vi "CLC_GEN3_L2_InPhaseCal.vi"() -> ()   [LabVIEW 2023, in "Clover_Cell.lvlib"]
uses:
  Clover_Cell.lvlib
  lib/Anritsu Signal Analyzer Series/Anritsu Signal Analyzer Series.lvlib
  lib/ELTA/ELTA.lvlib
  <vilib>/Utility/file.llb/Write Delimited Spreadsheet (DBL).vi
  <vilib>/Utility/file.llb/Write Delimited Spreadsheet (string).vi
panel:
  out "Check Ref. Ch.":i32[][](array[numeric])
  in  "Dual_Ch.???":bool=TRUE
  in  "Single_Channel_Phase_Sweep":bool
  in  "Polarity":u16(ring) items=["H", "V"]
  in  "AvgTimes":i32=3
  in  "TRXmode":u16(ring)=1 items=["Rx"=2, "Tx"=1]
  in  "CenterFreq(GHz)":dbl=27.0
  in  "VISA resource name":refnum<visa-resource-name>="TCPIP0::192.168.100.202::hislip0::INSTR"
  out "Channel":i32=63
  out "Operating \nChannel(s)":bool[][](array[boolean])
  out "FileNAME_Dual":string
  out "FileNAME_Single":string
  out "PhaseStep":i32=63
  out "OK?":bool
  out "output cluster":T1={"address"="192.168.100.111", "remote port or service name"=5025, "timeout ms (60000)"=10000}
  out "SA1":dbl[](graph)
  out "trmode":u16=1
  out "TotalTime":dbl format="%.2f"
  out "StopTime":timestamp=timestamp(3663835912.033212 s since 1904-01-01)
  out "Data":dbl[][](array[numeric])
  out "StartTime":timestamp=timestamp(3663835741.875155 s since 1904-01-01)
  out "error out":errorcluster
  out "CurrentData":dbl[](array[numeric])
  out "Duration":dbl
  # "CTTC Gen3 L2 8x8 in-Phase Calibration with SG/SA"
  # "Setting"
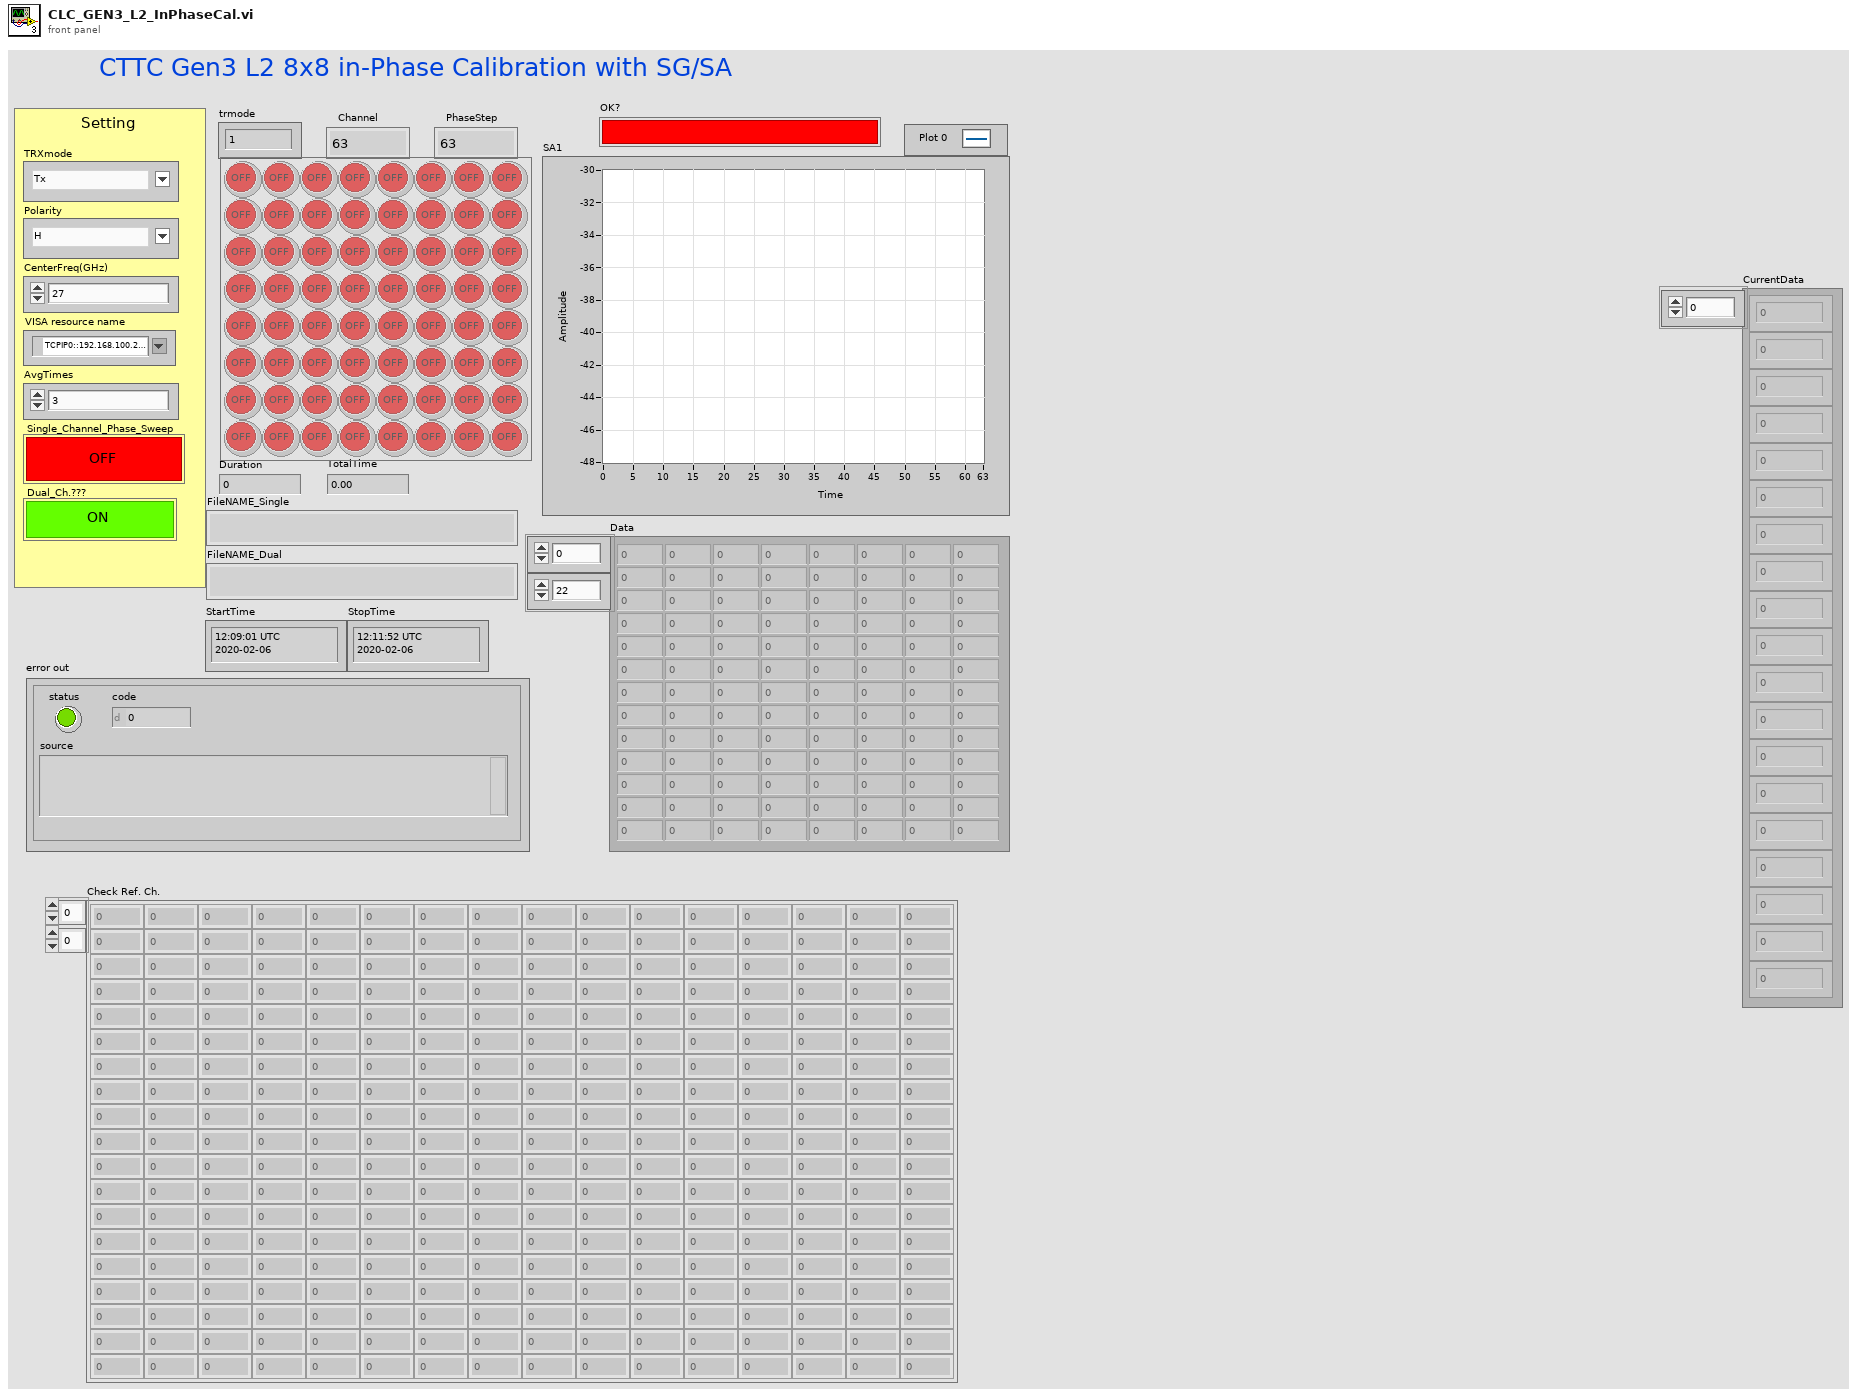
[diagram p1: front panel]
types:
  T1 = cluster{"address":string, "remote port or service name":u16, "timeout ms (60000)":i32}
  T2 = cluster{"Mode":u16, "Polarity":u16, "CH_ON/OFF":u16, "Channel":i32, "Gain":i32, "Phase":i32}
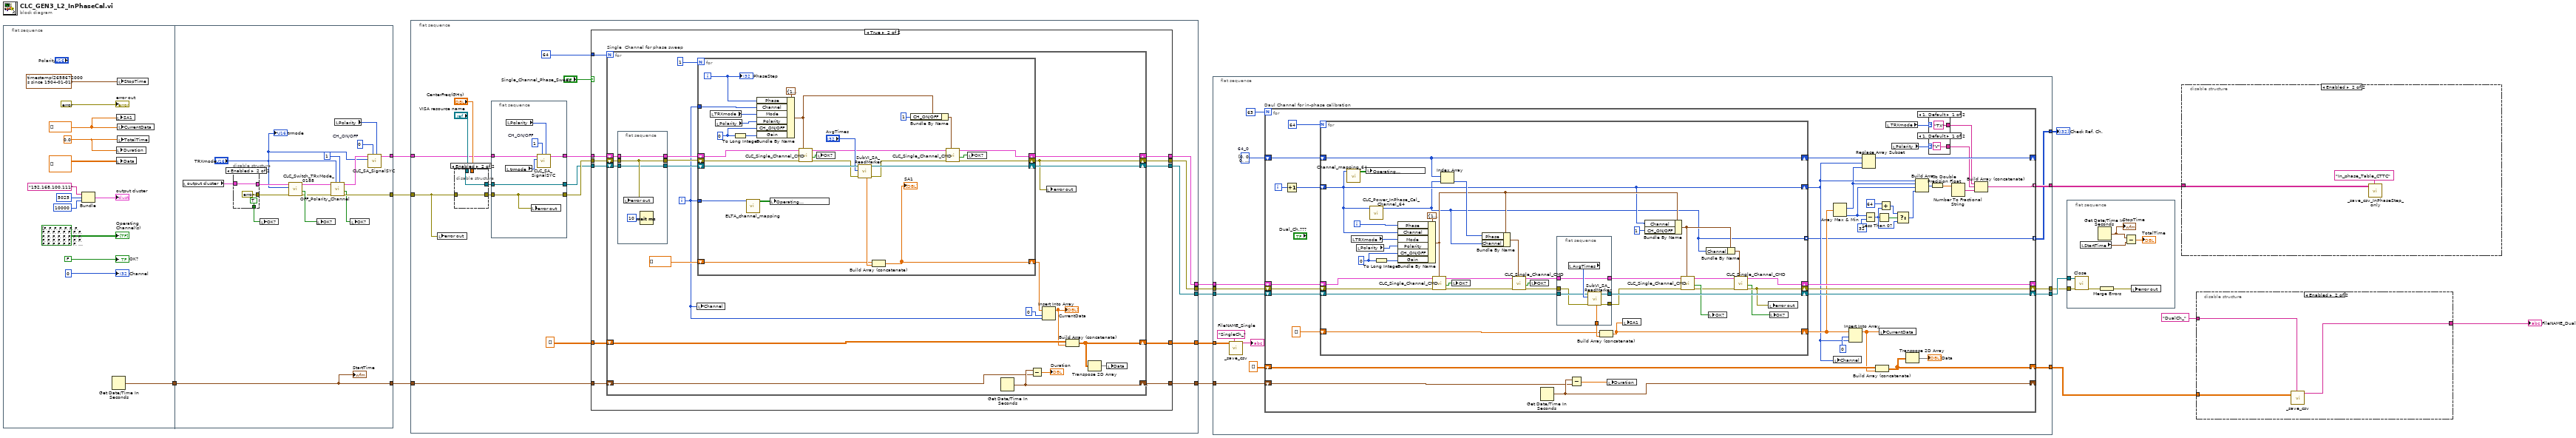
[diagram p0: block diagram]
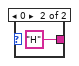
[diagram p2: hidden frame]
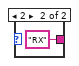
[diagram p3: hidden frame]
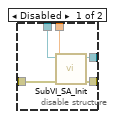
[diagram p4: hidden frame]
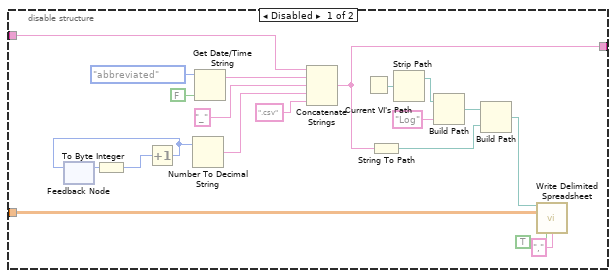
[diagram p6: hidden frame]
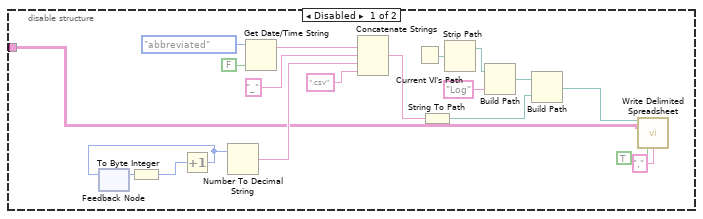
[diagram p7: hidden frame]
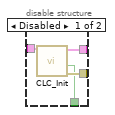
[diagram p8: hidden frame]
diagram:
  n1 = flat-sequence {
    tunnel: [w17] -> w4
    tunnel: w4 -> [w33]
    tunnel: [w36] -> w5
    tunnel: [w40] -> w6
    tunnel: [w33] -> w16
    frame #0 {
      w21 = dbl[] []
      w24 = 0.0 ("TotalTime")
      n2 = Bundle("address"="192.168.100.111", "remote port or service name"=u16 5025, "timeout ms (60000)"=10000) -> (→"output cluster":T1)  [unwired: 1 in]
      n3 = Get Date/Time In Seconds() -> (seconds since 1Jan1904=w17:timestamp)
      n4 = local write "SA1"(w21) -> ()
      n5 = local write "Duration"(w24) -> ()
      n6 = local write "Data"(dbl[][] []) -> ()
      n7 = local write "StopTime"(timestamp(2658672000.001 s since 1904-01-01) ("StopTime")) -> ()
      n8 = local write "CurrentData"(w21) -> ()
      n9 = local write "TotalTime"(w24) -> ()
      "error out" <- errorcluster {"status"=FALSE, "code"=0, "source"=""} ("error out")
      "Operating \nChannel(s)" <- bool[][] [[FALSE, FALSE, FALSE, FALSE, FALSE, FALSE, FALSE, FALSE], [FALSE, FALSE, FALSE, FALSE, FALSE, FALSE, FALSE, FALSE], [FALSE, FALSE, FALSE, FALSE, FALSE, FALSE, FALSE, FALSE], [FALSE, FALSE, FALSE, FALSE, FALSE, FALSE, FALSE, FALSE], [FALSE, FALSE, FALSE, FALSE, FALSE, FALSE, FALSE, FALSE], [FALSE, FALSE, FALSE, FALSE, FALSE, FALSE, FALSE, FALSE], [FALSE, FALSE, FALSE, FALSE, FALSE, FALSE, FALSE, FALSE], [FALSE, FALSE, FALSE, FALSE, FALSE, FALSE, FALSE, FALSE]] ("Operating \nChannel(s)")
      "Channel" <- 0 ("Channel")
      "OK?" <- FALSE ("OK?")
    }
    frame #1 {
      w35 = u16 0  # CH_ON/OFF
      n10 = local read "output cluster"() -> (w45:T1)
      n11 = disable-structure shown="Enabled" {
        disable-tunnel: w45 -> [w49 w52]
        disable-tunnel: [w48 w52] -> w44
        disable-tunnel: [w47 errorcluster {"status"=FALSE, "code"=0, "source"=""} ("error in (no error)")] -> w42
        disable-tunnel: [w46 TRUE ("OK?")] -> w34
        frame Disabled {
          n12 = call "CLC_Init.vi"("TCPIPin"=w49) -> ("error out"=w47:errorcluster, "Status"=w46:bool, "TCPIPin 2"=w48:T1)  [unwired: 8 in]
        }
        frame Enabled {
        }
      }
      n13 = local write "OK?"(w34) -> ()
      n14 = call "CLC_Switch_TRxMode_0188.vi"("error in (no error)"=w42, "Text Ring"="TRXmode", "TCPIPin"=w44) -> ("error out"=w41:errorcluster, "OK?"=w43:bool, "TCPIPin 2"=w39:T1)  [unwired: 6 in]
      n15 = local write "OK?"(w43) -> ()
      n16 = call "OFF_Polarity_Channel.vi"("CH_ON:0/OFF:1"=u16 1, "Mode"="TRXmode", "error in"=w41, "TCPIPin"=w39) -> ("error out"=w40:errorcluster, "OK?"=w38:bool, "TCPIPout"=w37:T1)  [unwired: 5 in]
      n17 = local read "Polarity"() -> (w31:u16)
      n18 = local write "OK?"(w38) -> ()
      n19 = call "CLC_SA_SignalSYC.vi"("Polarity"=w31, "CH_ON/OFF"=w35, "Mode"="TRXmode", "TCPIPin"=w37) -> ("TCPIPout"=w36:T1)  [unwired: 7 in]
      "StartTime" <- w33
      "trmode" <- "TRXmode"
    }
  }
  n20 = flat-sequence {
    tunnel: w16 -> [w68]
    tunnel: [w67] -> w15
    tunnel: [w66] -> w14
    tunnel: [w65] -> w13
    tunnel: [w64] -> w7
    tunnel: w6 -> [w62]
    tunnel: w5 -> [w58]
    tunnel: [w53] -> w3
    frame #0 {
      n21 = local write "error out"(w62) -> ()
      n22 = disable-structure shown="Enabled" {
        disable-tunnel: "VISA resource name" -> [w75 w76]
        disable-tunnel: [w74 w77] -> w63
        disable-tunnel: w62 -> [w73 w77]
        disable-tunnel: "CenterFreq(GHz)" -> [w72 _]
        disable-tunnel: [w71 w76] -> w57
        frame Disabled {
          n23 = call "SubVI_SA_Init.vi"("error in (no error)"=w73, "CenterFreq(GHz) 2"=w72, "VISA resource name"=w75) -> ("error out 2"=w74:errorcluster, "VISA resource name out"=w71:refnum<visa-resource-name>)  [unwired: 6 in, 1 out]
        }
        frame Enabled {
        }
      }
      n24 = flat-sequence {
        tunnel: w63 -> [w152]
        tunnel: [w152] -> w59
        tunnel: w58 -> [w150]
        tunnel: w57 -> [w151]
        tunnel: [w151] -> w56
        tunnel: [w149] -> w55
        frame #0 {
          w148 = u16 1  # CH_ON/OFF
          n25 = local read "trmode"() -> (w146:u16)
          n26 = local read "Polarity"() -> (w147:u16)
          n27 = local write "error out"(w152) -> ()
          n28 = call "CLC_SA_SignalSYC.vi"("Polarity"=w147, "CH_ON/OFF"=w148, "Mode"=w146, "TCPIPin"=w150) -> ("TCPIPout"=w149:T1)  [unwired: 7 in]
        }
      }
      n29 = case shown="True" "Single_Channel_Phase_Sweep" {
        tunnel: [w79 w93] -> w53
        tunnel: 64 -> [_ w92]
        tunnel: w68 -> [w78 w91]
        tunnel: [w80 w90] -> w67
        tunnel: [w81 w89] -> w66
        tunnel: [w82 w88] -> w65
        tunnel: [w78 w87] -> w64
        tunnel: dbl[][] [] -> [w79 w86]
        tunnel: w59 -> [w81 w85]
        tunnel: w56 -> [w80 w84]
        tunnel: w55 -> [w82 w83]
        frame False {
        }
        frame True {
          n30 = for "Single  Channel for phase sweep" {
            N: w92 -> [_]
            shift-right: [w114] -> w88
            shift-left: w83 -> [w99]
            shift-right: [w108] -> w89
            shift-left: w85 -> [w101]
            shift-right: [w112] -> w90
            shift-left: w84 -> [w98]
            shift-right: [w106] -> w93
            shift-left: w86 -> [w107]
            shift-right: [w110] -> w87
            shift-left: w91 -> [w109]
            i -> [w94]
            n31 = flat-sequence {
              tunnel: [w116] -> w97
              tunnel: w101 -> [w117]
              tunnel: [w117] -> w100
              tunnel: w99 -> [w116]
              tunnel: w98 -> [w115]
              tunnel: [w115] -> w96
              frame #0 {
                n32 = local write "error out"(w117) -> ()
                n33 = Wait (ms)(milliseconds to wait=u32 10) -> ()  [unwired: 1 out]
              }
            }
            n34 = local write "Channel"(w94) -> ()
            n35 = for {
              N: 1 -> [_]
              shift-right: [w125] -> w114
              shift-left: w97 -> [w137]
              shift-right: [w127] -> w108
              shift-left: w100 -> [w139]
              shift-right: [w144] -> w112
              shift-left: w96 -> [w145]
              shift-right: [w140] -> w105
              shift-left: dbl[] [] -> [w141]
              tunnel: w94 -> [w134]
              tunnel: w94 -> [w120]
              i -> [w130]
              w131 = u16 0 ("CH_ON/OFF")
              n36 = local read "TRXmode"() -> (w133:u16)
              n37 = local read "Polarity"() -> (w132:u16)
              n38 = To Long Integer(number=w131) -> (32bit integer=w129:i32)
              n39 = call "ELTA_channel_mapping.vi"("Channel IN"=w120) -> ("Operating \nChannel(s)"=w119:bool[][])  [unwired: 10 in]
              n40 = Bundle By Name(cluster=T2 {"Mode"=1, "Polarity"=1, "CH_ON/OFF"=1, "Channel"=0, "Gain"=0, "Phase"=0} ("Channel params"), "Phase"=w130, "Channel"=w134, "Mode"=w133, "Polarity"=w132, "CH_ON/OFF"=w131, "Gain"=w129) -> (w124:T2)
              n41 = local write "Operating \nChannel(s)"(w119) -> ()
              n42 = call "CLC_Single_Channel_CMD.vi"("Channel params"=w124, "error in"=w139, "TCPIPin"=w137) -> ("error out"=w138:errorcluster, "OK?"=w135:bool, "TCPIPout"=w126:T1)  [unwired: 6 in]
              n43 = local write "OK?"(w135) -> ()
              n44 = call "SubVI_SA_ReadMarker.vi"("error in (no error)"=w138, "AvgTimes"="AvgTimes", "VISA resource name"=w145) -> ("error out"=w128:errorcluster, "VISA resource name out"=w144:refnum<visa-resource-name>, "Marker Power"=w142:dbl)  [unwired: 5 in, 1 out]
              n45 = Build Array (concatenate)(w141, w142) -> (w140:dbl[])
              "SA1" <- w140
              n46 = Bundle By Name(cluster=w124, "CH_ON/OFF"=u16 1) -> (w122:T2)
              n47 = call "CLC_Single_Channel_CMD.vi"("Channel params"=w122, "error in"=w128, "TCPIPin"=w126) -> ("error out"=w127:errorcluster, "OK?"=w121:bool, "TCPIPout"=w125:T1)  [unwired: 6 in]
              n48 = local write "OK?"(w121) -> ()
              "PhaseStep" <- w130
            }
            n49 = Get Date/Time In Seconds() -> (seconds since 1Jan1904=w110:timestamp)
            n50 = Subtract(x=w110, y=w109) -> (x-y=→"Duration":dbl)
            n51 = Insert Into Array(array=w105, index=0, new element=w94) -> (w103:dbl[])
            "CurrentData" <- w103
            n52 = local write "error out"(w108) -> ()
            n53 = Build Array (concatenate)(w107, w103) -> (w106:dbl[][])
            n54 = Transpose 2D Array(2D array=w106) -> (transposed array=w95:dbl[][])
            n55 = local write "Data"(w95) -> ()
          }
        }
      }
    }
  }
  n56 = flat-sequence {
    tunnel: w15 -> [w166]
    tunnel: w14 -> [w165]
    tunnel: w13 -> [w164]
    tunnel: [w163] -> w10
    tunnel: [w162] -> w9
    tunnel: [w161] -> w8
    tunnel: w7 -> [w160]
    tunnel: [w158] -> w1
    tunnel: w3 -> [w157]
    tunnel: [w153] -> w2
    frame #0 {
      w154 = i32[] [0, 0, 0, 0, 0, 0, 0, 0, 0, 0, 0, 0, 0, 0, 0, 0, 0, 0, 0, 0, 0, 0, 0, 0, 0, 0, 0, 0, 0, 0, 0, 0, 0, 0, 0, 0, 0, 0, 0, 0, 0, 0, 0, 0, 0, 0, 0, 0, 0, 0, 0, 0, 0, 0, 0, 0, 0, 0, 0, 0, 0, 0, 0, 0]  # 64_0
      n57 = call "_save_csv.vi"("delimiter (\\t)"="SingleCh_" ("delimiter (\\t)"), "Data"=w157) -> ("FileName"=→"FileNAME_Single":string)  [unwired: 9 in]
      n58 = for "Daul Channel for in-phase calibration" {
        N: 63 -> [_]
        shift-right: [w207] -> _
        shift-left: w164 -> [w192]
        shift-right: [w204] -> w161
        shift-left: w165 -> [w193]
        shift-right: [w205] -> w162
        shift-left: w166 -> [w203]
        shift-right: [w198] -> w163
        shift-left: dbl[][] [] -> [w199]
        shift-right: [w202] -> _
        shift-left: w160 -> [w201]
        shift-right: [w181] -> _
        shift-left: w154 -> [w190]
        tunnel: [w168] -> w158 mode=indexing
        tunnel: [w178] -> w153 mode=indexing
        i -> [w177]
        n59 = Increment(x=w177) -> (x+1=w176:i32)
        n60 = for {
          N: 64 -> [_]
          shift-right: [w217] -> w207
          shift-left: w192 -> [w237]
          shift-right: [w222] -> w204
          shift-left: w193 -> [w239]
          shift-right: [w248] -> w205
          shift-left: w203 -> [w245]
          shift-right: [w214] -> w191
          shift-left: dbl[] [] -> [w246]
          shift-right: [w230] -> w182
          shift-left: w190 -> [w230]
          shift-right: [w213] -> w179
          shift-left: w176 -> [w213]
          tunnel: [w212] -> w178 mode=indexing
          i -> [w238]
          w243 = u16 0 ("CH_ON/OFF")
          n61 = call "Channel_mapping_64.vi"("Channel IN"=w213) -> ("Operating \nChannel(s)"=w216:bool[][])  [unwired: 10 in]
          n62 = local read "TRXmode"() -> (w241:u16)
          n63 = local read "Polarity"() -> (w242:u16)
          n64 = local write "Operating \nChannel(s)"(w216) -> ()
          n65 = call "CLC_Power_InPhase_Cal_Channel_64.vi"("Channel IN"=w213) -> ("Ref_Channel"=w212:i32)  [unwired: 8 in, 2 out]
          n66 = To Long Integer(number=w243) -> (32bit integer=w244:i32)
          n67 = Bundle By Name(cluster=T2 {"Mode"=1, "Polarity"=1, "CH_ON/OFF"=1, "Channel"=0, "Gain"=0, "Phase"=0} ("Channel params"), "Phase"=w238, "Channel"=w213, "Mode"=w241, "Polarity"=w242, "CH_ON/OFF"=w243, "Gain"=w244) -> (w220:T2)
          n68 = call "CLC_Single_Channel_CMD.vi"("Channel params"=w220, "error in"=w239, "TCPIPin"=w237) -> ("error out"=w235:errorcluster, "OK?"=w234:bool, "TCPIPout"=w236:T1)  [unwired: 6 in]
          n69 = Index Array(array=w230, index=w212) -> (element=w229:i32)
          n70 = local write "OK?"(w234) -> ()
          n71 = Bundle By Name(cluster=w220, "Phase"=w229, "Channel"=w212) -> (w233:T2)
          n72 = call "CLC_Single_Channel_CMD.vi"("Channel params"=w233, "error in"=w235, "TCPIPin"=w236) -> ("error out"=w231:errorcluster, "OK?"=w232:bool, "TCPIPout"=w228:T1)  [unwired: 6 in]
          n73 = local write "OK?"(w232) -> ()
          n74 = flat-sequence {
            tunnel: [w255] -> w248
            tunnel: [w253] -> w247
            tunnel: [w252] -> w227
            tunnel: w245 -> [w251]
            tunnel: w231 -> [w250]
            tunnel: [w249] -> w226
            tunnel: w228 -> [w249]
            frame #0 {
              n75 = local read "AvgTimes"() -> (w254:i32)
              n76 = call "SubVI_SA_ReadMarker.vi"("error in (no error)"=w250, "AvgTimes"=w254, "VISA resource name"=w251) -> ("error out"=w252:errorcluster, "VISA resource name out"=w255:refnum<visa-resource-name>, "Marker Power"=w253:dbl)  [unwired: 5 in, 1 out]
            }
          }
          n77 = Build Array (concatenate)(w246, w247) -> (w214:dbl[])
          n78 = local write "SA1"(w214) -> ()
          n79 = Bundle By Name(cluster=w220, "Channel"=w213, "CH_ON/OFF"=u16 1) -> (w215:T2)
          n80 = call "CLC_Single_Channel_CMD.vi"("Channel params"=w215, "error in"=w227, "TCPIPin"=w226) -> ("error out"=w223:errorcluster, "OK?"=w224:bool, "TCPIPout"=w221:T1)  [unwired: 6 in]
          n81 = Bundle By Name(cluster=w215, "Channel"=w212) -> (w219:T2)
          n82 = local write "OK?"(w224) -> ()
          n83 = call "CLC_Single_Channel_CMD.vi"("Channel params"=w219, "error in"=w223, "TCPIPin"=w221) -> ("error out"=w222:errorcluster, "OK?"=w218:bool, "TCPIPout"=w217:T1)  [unwired: 6 in]
          n84 = local write "error out"(w222) -> ()
          n85 = local write "OK?"(w218) -> ()
        }
        n86 = Get Date/Time In Seconds() -> (seconds since 1Jan1904=w202:timestamp)
        n87 = Subtract(x=w202, y=w201) -> (x-y=w200:dbl)
        n88 = local write "Duration"(w200) -> ()
        n89 = Array Max & Min(array=w191) -> (max index (indices)=w180:i32, min index (indices)=w189:i32)  [unwired: 2 out]
        n90 = local write "Channel"(w179) -> ()
        n91 = Insert Into Array(array=w191, index=0, new element=w179) -> (w194:dbl[])
        n92 = Replace Array Subset(array=w182, new element=w180, index=w179) -> (w181:i32[])
        n93 = Subtract(x=w189, y=32) -> (x-y=w184:i32)
        n94 = Build Array (concatenate)(w199, w194) -> (w198:dbl[][])
        n95 = Less Than 0?(x=w184) -> (x < 0?=w187:bool)
        n96 = Add(x=64, y=w184) -> (x+y=w185:i32)
        n97 = local write "CurrentData"(w194) -> ()
        n98 = local read "TRXmode"() -> (w171:u16)
        n99 = local read "Polarity"() -> (w172:u16)
        n100 = Select(t=w185, s=w187, f=w184) -> (s? t:f=w183:i32)
        n101 = Transpose 2D Array(2D array=w198) -> (transposed array=→"Data":dbl[][])
        n102 = Build Array(w179, w180, w189, w183) -> (w175:i32[])
        n103 = case shown="1, Default" w171 {
          tunnel: ["TX" "RX"] -> w169
          frame 1, Default {
          }
          frame 2 {
          }
        }
        n104 = case shown="1, Default" w172 {
          tunnel: ["V" "H"] -> w170
          frame 1, Default {
          }
          frame 0 {
          }
        }
        n105 = To Double Precision Float(number=w175) -> (double precision float=w174:dbl[])
        n106 = Number To Fractional String(number=w174) -> (F-format string=w173:string[])  [unwired: 3 in]
        n107 = Build Array (concatenate)(w169, w170, w173) -> (w168:string[])
      }
    }
  }
  n108 = flat-sequence {
    tunnel: w9 -> [w261]
    tunnel: w8 -> [w260]
    frame #0 {
      n109 = call "Close.vi"("error in (no error)"=w260, "VISA resource name"=w261) -> ("error out"=w262:errorcluster)  [unwired: 9 in]
      n110 = local read "StartTime"() -> (w256:timestamp)
      n111 = Get Date/Time In Seconds() -> (seconds since 1Jan1904=w257:timestamp)
      "StopTime" <- w257
      n112 = Merge Errors(w262) -> (w259:errorcluster)
      n113 = Subtract(x=w257, y=w256) -> (x-y=→"TotalTime":dbl)
      n114 = local write "error out"(w259) -> ()
    }
  }
  n115 = disable-structure shown="Enabled" {
    disable-tunnel: w1 -> [w264 w283]
    frame Disabled {
      n116 = feedback #1() -> (w273:i8)  [unwired: 1 in]
      n117 = To Byte Integer(number=w273) -> (8bit integer=w275:i8)
      n118 = Increment(x=w275) -> (x+1=w274:i8)
      n119 = feedback-in #1(w274) -> ()
      n120 = Number To Decimal String(number=w274) -> (decimal integer string=w276:string)  [unwired: 1 in]
      n121 = Get Date/Time String(date format (0)=enum16{"short", "long", "abbreviated"}."abbreviated", want seconds? (F)=FALSE) -> (date string=w267:string)  [unwired: 1 in, 1 out]
      n122 = Concatenate Strings(w267, "_" ("delimiter (\\t)"), w276, ".csv" ("delimiter (\\t)")) -> (w268:string, w272:string)
      n123 = Current VI's Path() -> (path=w281:path)
      n124 = String To Path(string=w268) -> (path=w282:path)
      n125 = Strip Path(path=w281) -> (stripped path=w280:path)  [unwired: 1 out]
      n126 = Build Path(base path=w280, name or relative path="Log") -> (appended path=w278:path)
      n127 = Build Path(base path=w278, name or relative path=w282) -> (appended path=w263:path)
      n128 = call-poly <vilib>:"Write Delimited Spreadsheet.vi"("file path (dialog if empty)"=w263, "2D data"=w264, "transpose? (no:F)"=TRUE, "delimiter (\\t)"="," ("delimiter (\\t)")) -> ()  [unwired: 10 in, 2 out]
    }
    frame Enabled {
      n129 = call "_save_csv_InPhaseStep_only.vi"("delimiter (\\t)"="In_phase_Table_CTTC" ("delimiter (\\t)"), "dataInput"=w283) -> ()  [unwired: 9 in, 1 out]
    }
  }
  n130 = disable-structure shown="Enabled" {
    disable-tunnel: [w303 w305] -> w12
    disable-tunnel: "DualCh_" ("delimiter (\\t)") -> [w299 w306]
    disable-tunnel: w10 -> [w298 w307]
    frame Disabled {
      n131 = feedback #2() -> (w297:i8)  [unwired: 1 in]
      n132 = To Byte Integer(number=w297) -> (8bit integer=w295:i8)
      n133 = Increment(x=w295) -> (x+1=w296:i8)
      n134 = feedback-in #2(w296) -> ()
      n135 = Number To Decimal String(number=w296) -> (decimal integer string=w294:string)  [unwired: 1 in]
      n136 = Get Date/Time String(date format (0)=enum16{"short", "long", "abbreviated"}."abbreviated", want seconds? (F)=FALSE) -> (date string=w304:string)  [unwired: 1 in, 1 out]
      n137 = Concatenate Strings(w299, w304, "_" ("delimiter (\\t)"), w294, ".csv" ("delimiter (\\t)")) -> (w303:string)
      n138 = Current VI's Path() -> (path=w289:path)
      n139 = String To Path(string=w303) -> (path=w288:path)
      n140 = Strip Path(path=w289) -> (stripped path=w290:path)  [unwired: 1 out]
      n141 = Build Path(base path=w290, name or relative path="Log") -> (appended path=w292:path)
      n142 = Build Path(base path=w292, name or relative path=w288) -> (appended path=w287:path)
      n143 = call-poly <vilib>:"Write Delimited Spreadsheet.vi"("file path (dialog if empty)"=w287, "2D data"=w298, "transpose? (no:F)"=TRUE, "delimiter (\\t)"="," ("delimiter (\\t)")) -> ()  [unwired: 10 in, 2 out]
    }
    frame Enabled {
      n144 = call "_save_csv.vi"("delimiter (\\t)"=w306, "Data"=w307) -> ("FileName"=w305:string)  [unwired: 9 in]
    }
  }
  "FileNAME_Dual" <- w12
  "Check Ref. Ch." <- w2
